vi "Get Version.vi"(8 "error in (no error)":errorcluster, 11 "Core Configurations in":refnum<class "Core Component Configurations.lvclass">) -> (0 "error out":errorcluster, 2 "version":T1, 3 "Core Configurations out":refnum<class "Core Component Configurations.lvclass">)   [LabVIEW 2019, in "DSF Core.lvlib" / "Core Component Configurations.lvclass"]
uses:
  Core Component Configurations.lvclass
  Typedefs/DSF Version Info.ctl
  DSF Core.lvlib
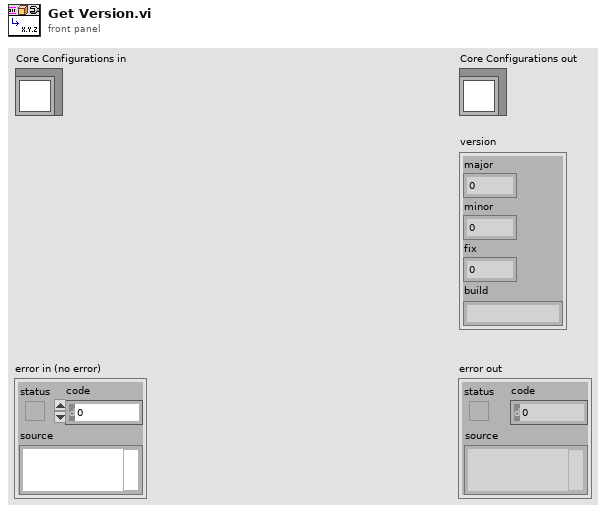
[diagram p1: front panel]
types:
  T1 = typedef "DSF Core.lvlib/DSF Version Info.ctl" = cluster{"major":u32, "minor":u32, "fix":u32, "build":string}
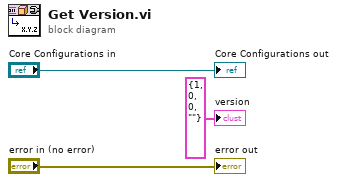
[diagram p0: block diagram]
diagram:
  "error out" <- "error in (no error)"
  "Core Configurations out" <- "Core Configurations in"
  "version" <- T1 {"major"=1, "minor"=0, "fix"=0, "build"=""} ("version")
